vi "Convert Description To Cluster.vi"(8 "Description String (empty)":string, 9 "error in (no error)":errorcluster) -> (0 "Description Cluster":T1, 1 "error out":errorcluster)   [LabVIEW 2014]
doc: "<b>VI Description:</b> This VI expands the documentation (description) string of a VI into separate fields based on the control label names. \n<b>VI Version:</b> 1.0.40.beta \n<b>Review Date:</b> 03/09/2012 \n<b>Author:</b> Jason Willis, Ryan Podsim \n<b>Copyright:</b> Copyright © 2010-2014"
uses:
  TYPE_Description Cluster.ctl
  TYPE_Version Status.ctl
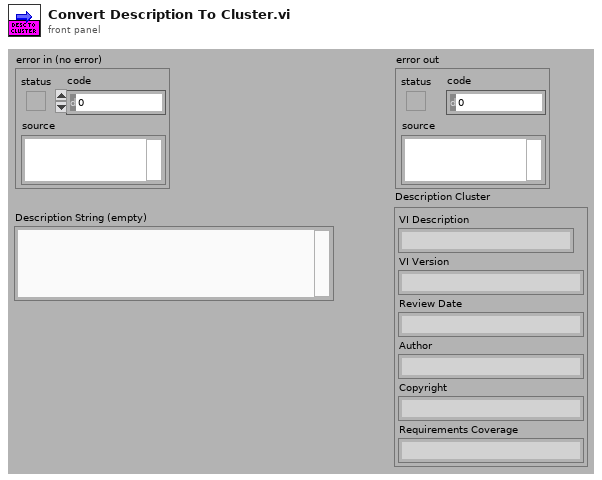
[diagram p1: front panel]
types:
  T1 = typedef "TYPE_Description Cluster.ctl" = cluster{"VI Description":string, "VI Version":string, "Review Date":string, "Author":string, "Copyright":string, "Requirements Coverage":string}
  T2 = typedef "TYPE_Version Status.ctl" = enum16{"Development", "alpha", "beta", "Reviewed", "Bug", "Other"}
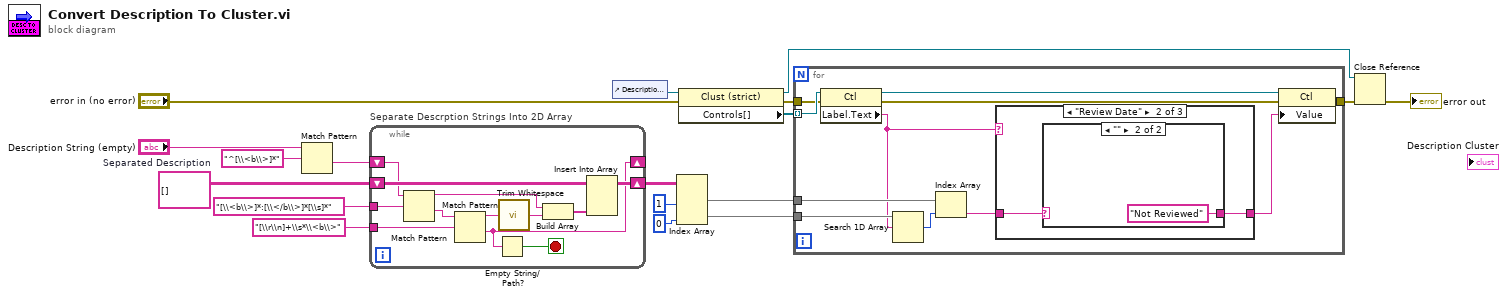
[diagram p0: block diagram]
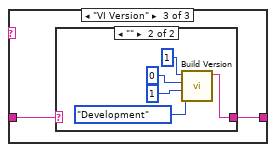
[diagram p4: hidden frame]
diagram:
  w11 = string[][] []  # Separated Description
  n1 = Match Pattern(string="Description String (empty)", regular expression="^[\\<b\\>]*" ("Author")) -> (after substring=w3:string)  [unwired: 1 in, 3 out]
  n2 = while "Separate Descrption Strings Into 2D Array" {
    shift-right: [w21] -> _
    shift-left: w3 -> [w23]
    shift-right: [w28] -> w8
    shift-left: w11 -> [w29]
    tunnel: "[\\<b\\>]*:[\\</b\\>]*[\\s]*" ("Author") -> [w25]
    tunnel: "[\\r\\n]+\\s*\\<b\\>" ("Author") -> [w24]
    stop <- w30 stop-if-true
    n3 = Match Pattern(string=w23, regular expression=w25) -> (before substring=w27:string, after substring=w26:string)  [unwired: 1 in, 2 out]
    n4 = Match Pattern(string=w26, regular expression=w24) -> (before substring=w19:string, after substring=w21:string)  [unwired: 1 in, 2 out]
    n5 = Empty String/Path?(string/path=w21) -> (empty?=w30:bool)
    n6 = call <vilib>:"Trim Whitespace.vi"("string"=w19) -> ("trimmed string"=w20:string)  [unwired: 1 in]
    n7 = Build Array(w27, w20) -> (w22:string[])
    n8 = Insert Into Array(array=w29, new element=w22) -> (w28:string[][])  [unwired: 2 in]
  }
  n9 = control-ref of="Description Cluster"() -> (w12:refnum<vi>)
  n10 = Index Array(array=w8, index (col) #1=1 ("disabled index (col)"), index (col) #2=0 ("disabled index (col)")) -> (element #1=w2:string[], element #2=w1:string[])  [unwired: 2 in]
  n11 = property class="Clust (strict)"(reference=w12, error in="error in (no error)") -> (reference out=w13:refnum<vi>, error out=w15:errorcluster, "Controls[]"=w16:refnum<vi>[])
  n12 = for {
    tunnel: w16 -> [w41] mode=indexing
    tunnel: w1 -> [w34]
    tunnel: w2 -> [w35]
    tunnel: w15 -> [w37]
    tunnel: [w36] -> w14
    n13 = property class="Ctl"(reference=w41, error in=w37) -> (reference out=w39:refnum<vi>, error out=w38:errorcluster, "Label.Text"=w33:string)
    n14 = Search 1D Array(1D array=w34, element=w33) -> (index of element=w40:i32)  [unwired: 1 out]
    n15 = Index Array(array=w35, index=w40) -> (element=w32:string)
    n16 = case shown="\"Review Date\"" w33 {
      tunnel: [w42 w44 w48] -> w31
      tunnel: w32 -> [w42 w43 w47]
      frame Default {
      }
      frame "Review Date" {
        n17 = case shown="\"\"" w43 {
          selector: w43 -> [w45 _]
          tunnel: [w45 "Not Reviewed"] -> w44
          frame Default {
          }
          frame "" {
          }
        }
      }
      frame "VI Version" {
        n18 = case shown="\"\"" w47 {
          selector: w47 -> [w49 _]
          tunnel: [w49 w53] -> w48
          frame Default {
          }
          frame "" {
            n19 = call "Build Version.vi"("Current Phase"=TYPE_Version_Status."Development", "Revision"=u32 1, "Minor Revision"=u16 0, "Major Revision"=u16 1) -> ("VI Version"=w53:string)  [unwired: 7 in]
          }
        }
      }
    }
    n20 = property class="Ctl"(reference=w39, error in=w38, "Value"=w31) -> (error out=w36:errorcluster)  [unwired: 1 out]
  }
  n21 = Close Reference(reference=w13, error in (no error)=w14) -> (error out=→"error out":errorcluster)
